vi "Pre Launch Init.vi"(11 "Task Viewer in":refnum<class "Task Viewer.lvclass">) -> (0 "error out":errorcluster, 3 "Task Viewer out":refnum<class "Task Viewer.lvclass">)   [LabVIEW 2020, in "Task Viewer.lvlib" / "Task Viewer.lvclass"]
doc: "Initializes the panel actor. Creates the Panel Helper.\n\n----\nPlease see the following web address for additional documentation and tutorial information:\nhttp://www.mooregoodideas.com/mgi-panel-manager/\n\nAuthor: Derek Trepanier\n\nCopyright (c) 2018, Moore Good Ideas, Inc.\n\nAll rights reserved.\n\nRedistribution and use in source and binary forms, with or without modification, are permitted provided that the following conditions are met:\n\n * Redistributions of source code must retain the above copyright notice, this list of conditions and the following disclaimer.\n * Redistributions in binary form must reproduce the above copyright notice, this list of conditions and the following disclaimer in the documentation and/or other materials provided with the distribution.\n * Neither the name of Moore Good Ideas, Inc. nor the names of its contributors may be used to endorse or promote products derived from this software without specific prior written permission.\n\nTHIS SOFTWARE IS PROVIDED BY THE COPYRIGHT HOLDERS AND CONTRIBUTORS \"AS IS\" AND ANY EXPRESS OR IMPLIED WARRANTIES, INCLUDING, BUT NOT LIMITED TO, THE IMPLIED WARRANTIES OF MERCHANTABILITY AND FITNESS FOR A PARTICULAR PURPOSE ARE DISCLAIMED. IN NO EVENT SHALL THE COPYRIGHT OWNER OR CONTRIBUTORS BE LIABLE FOR ANY DIRECT, INDIRECT, INCIDENTAL, SPECIAL, EXEMPLARY, OR CONSEQUENTIAL DAMAGES (INCLUDING, BUT NOT LIMITED TO, PROCUREMENT OF SUBSTITUTE GOODS OR SERVICES; LOSS OF USE, DATA, OR PROFITS; OR BUSINESS INTERRUPTION) HOWEVER CAUSED AND ON ANY THEORY OF LIABILITY, WHETHER IN CONTRACT, STRICT LIABILITY, OR TORT (INCLUDING NEGLIGENCE OR OTHERWISE) ARISING IN ANY WAY OUT OF THE USE OF THIS SOFTWARE, EVEN IF ADVISED OF THE POSSIBILITY OF SUCH DAMAGE."
uses:
  Task Viewer.lvclass
  Task Viewer enum df.ctl
  Task Viewer.lvclass/Task Viewer.ctl
  <vilib>/MGI/Panel Manager/Panel Actor/Panel Actor/Panel Actor.lvclass
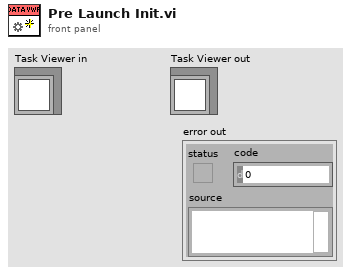
[diagram p1: front panel]
types:
  T1 = typedef "Task Viewer enum df.ctl" = enum16{"Idle", "Countdown", "Close Helper"}
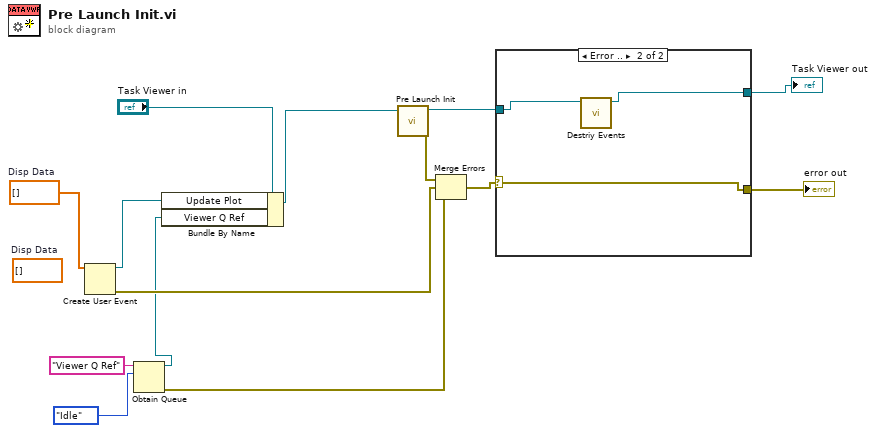
[diagram p0: block diagram]
diagram:
  w1 = dbl[] []  # Disp Data
  (unwired) dbl[] []  # Disp Data
  n1 = Create User Event(user event datatype=w1) -> (user event=w6:refnum<user-event>, error out=w7:errorcluster)  [unwired: 1 in]
  n2 = Obtain Queue(name (unnamed)="Viewer Q Ref", element data type=Task_Viewer_enum_df."Idle") -> (queue out=w2:refnum<queue>, error out=w4:errorcluster)  [unwired: 3 in, 1 out]
  n3 = Bundle By Name(cluster="Task Viewer in", "Update Plot"=w6, "Viewer Q Ref"=w2) -> (w8:refnum<class "Task Viewer.lvclass">)
  n4 = call-parent "Pre Launch Init.vi"("Panel Actor in"=w8) -> ("error out"=w11:errorcluster, "Panel Actor out"=w13:refnum<class "Task Viewer.lvclass">)  [unwired: 9 in]
  n5 = Merge Errors(w11, w7, w4) -> (w12:errorcluster)
  n6 = case shown="Error .." w12 {
    selector: w12 -> [w15 w19]
    tunnel: [w16 w17] -> w14
    tunnel: w13 -> [w16 w18]
    tunnel: [w15 w19] -> w10
    frame No Error {
    }
    frame Error {
      n7 = call "Destriy Events.vi"("Task Viewer in"=w18) -> ("Task Viewer out"=w17:refnum<class "Task Viewer.lvclass">)  [unwired: 9 in, 1 out]
    }
  }
  "error out" <- w10
  "Task Viewer out" <- w14
